vi "Write Numeric data.vi"(8 "error in (no error)":errorcluster, 10 "Numeric data":dbl, 11 "Communication in":refnum<class "Communication.lvclass">) -> (0 "error out":errorcluster, 3 "Communication out":refnum<class "Communication.lvclass">)   [LabVIEW 2020, in "Communication.lvclass"]
uses:
  Communication.lvclass
  Communication.lvclass/Communication.ctl
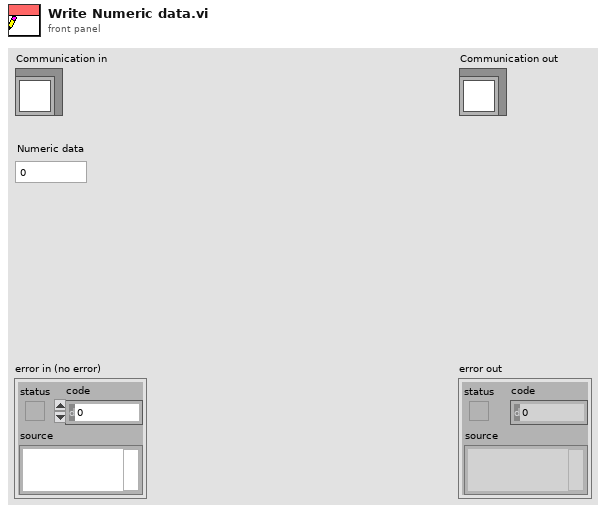
[diagram p1: front panel]
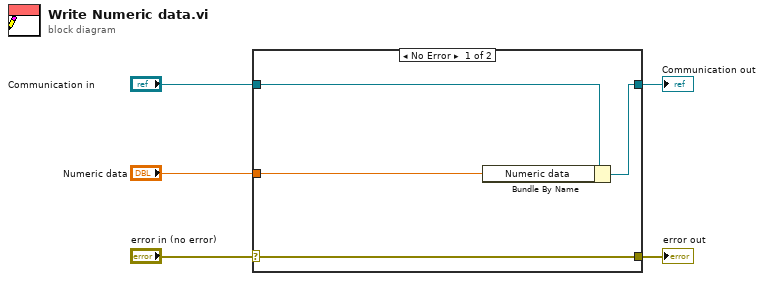
[diagram p0: block diagram]
diagram:
  n1 = case shown="No Error" "error in (no error)" {
    selector: "error in (no error)" -> [w9 w10]
    tunnel: [w9 w10] -> w4
    tunnel: [w7 w11] -> w2
    tunnel: "Communication in" -> [w8 w11]
    tunnel: "Numeric data" -> [w6 _]
    frame No Error {
      n2 = Bundle By Name(cluster=w8, "Numeric data"=w6) -> (w7:refnum<class "Communication.lvclass">)
    }
    frame Error {
    }
  }
  "error out" <- w4
  "Communication out" <- w2
